vi "Tim Horizontal Bearing Control.vi"() -> ()   [LabVIEW 2020]
doc: "I. Description:\nThis example demonstrates how to output a single Voltage Update (Sample) to an Analog Output Channel.\n\nII. Instructions for Running:\n1. Select the Physical Channel to correspond to where your signal is output on the DAQ device.\n2. Enter the Minimum and Maximum Voltage Ranges\nNote: Use the Acq One Sample example to verify you are generating the correct output on the DAQ device\n\nIII. Block Diagram Steps:\n1. Create an Analog Output Voltage Channel\n2. Use the Write VI to Output 1 Sample to 1 Channel on the Data\nAcquisition Card. \n3. Call the Clear Task VI to clear the Task.\n4. Use the popup dialog box to display an error if any. \n\nIV. I/O Connections Overview:\nMake sure your signal output terminal matches the Physical Channel I/O Control. For further connection information, refer to your hardware reference manual."
uses:
  <vilib>/DAQmx/write.llb/DAQmx Write (Digital Bool 1Line 1Point).vi
  <vilib>/DAQmx/read.llb/DAQmx Read (Counter DBL 1Chan 1Samp).vi
  <extravilib>/ChannelInstances/Tag-bool/Write With Abort.vi
  <extravilib>/ChannelInstances/Tag-bool/Read With Abort.vi
  <extravilib>/ChannelInstances/Tag-dbl/Write With Abort.vi
  <extravilib>/ChannelInstances/Tag-dbl/Read With Abort.vi
  <vilib>/DAQmx/create/channels.llb/DAQmx Create Channel (CI-Frequency).vi
  <vilib>/DAQmx/configure/timing.llb/DAQmx Timing (Implicit).vi
  <vilib>/DAQmx/create/channels.llb/DAQmx Create Channel (DO-Digital Output).vi
  <extravilib>/ChannelInstances/Tag-bool/Instantiate.vi
  <extravilib>/ChannelInstances/Messenger-c(str,a[.](str),var)/Instantiate.vi
  <extravilib>/ChannelInstances/Tag-bool/Endpoint.vi
  <extravilib>/ChannelInstances/Tag-bool/EndpointRead.vi
  <extravilib>/ChannelInstances/Tag-dbl/Instantiate.vi
  <vilib>/DAQmx/miscellaneous.llb/DAQmx Fill In Error Info.vi
  <extravilib>/ChannelInstances/Tag-dbl/Endpoint.vi
  Labview_dependencies/channel_producer_dbl.vi
  <extravilib>/ChannelInstances/Tag-dbl/EndpointRead.vi
  <extravilib>/ChannelInstances/Tag-dbl.lvlib
  <extravilib>/ChannelInstances/Tag-bool.lvlib
  <resource>/objmgr/daqmx.rc
panel:
  in  "Relay":tag="cDAQ9189-horizontalMod7/port0/line5"
  in  "TCPIP Socket":refnum<visa-resource-name>="TCPIP0::10.0.0.52::5000::SOCKET"
  in  "CL Frequency Term":tag="/cDAQ9189-horizontalMod7/PFI0"
  in  "Counter":tag="cDAQ9189-horizontalMod7/ctr0"
  out "RPM":dbl
  in  "Toggle":bool
  in  "stop":bool
  in  "Save Folder":path
  in  "Save 2":bool
  out "Temp 1":dbl format="%.3f"
  out "Temp 2":dbl format="%.3f"
  out "Temp 3":dbl format="%.3f"
  out "Temp 4":dbl format="%.3f"
  out "Waveform Graph":dbl[][](graph)
  # "Physical Connections"
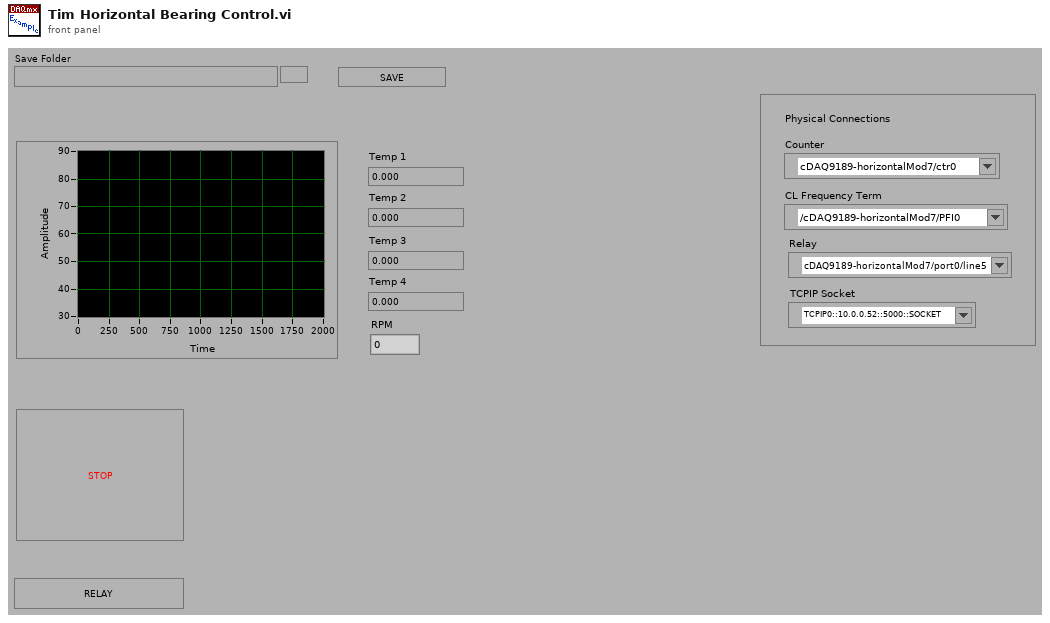
[diagram p1: front panel]
types:
  T1 = enum16{"open", "open or create", "create or replace", "create", "open (read-only)"}
  T2 = typedef "Tag-bool.lvlib/))Channel.ctl" = refnum<queue>
  T3 = typedef "Tag-dbl.lvlib/))Channel.ctl" = refnum<queue>
  T4 = typedef "Messenger-c(str,a[.](str),var).lvlib/))Channel.ctl" = refnum<queue>
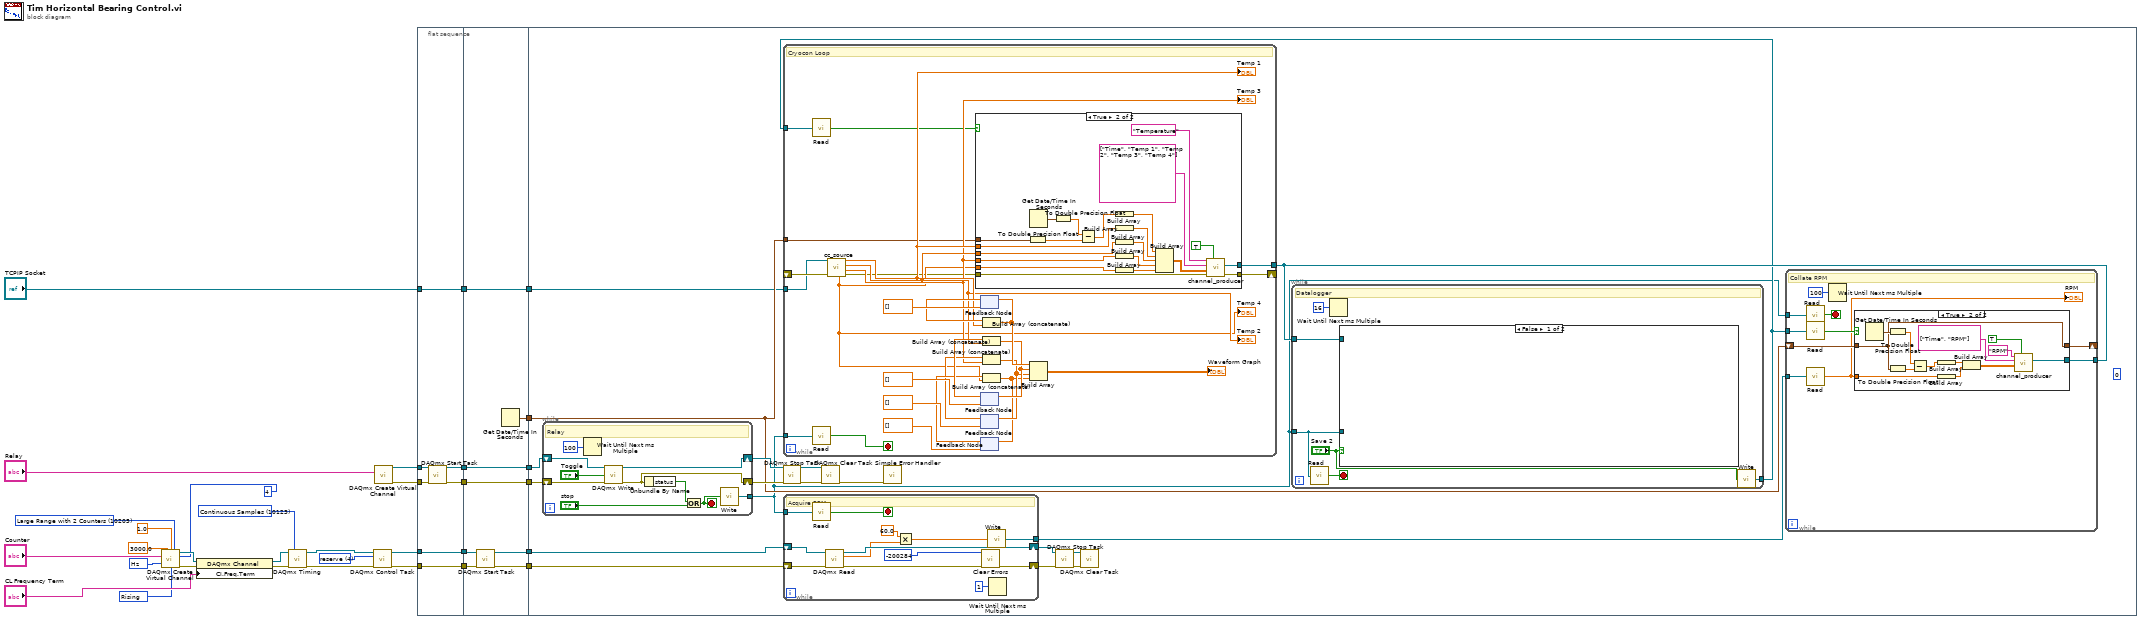
[diagram p0: block diagram]
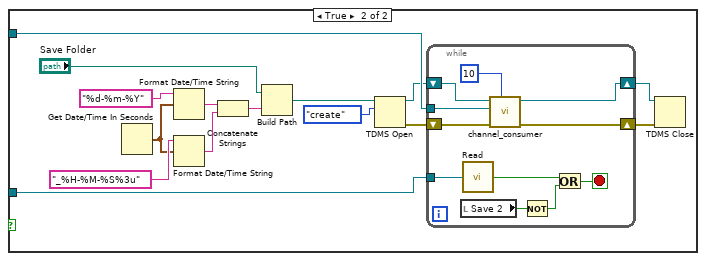
[diagram p3: hidden frame]
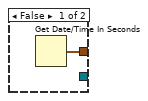
[diagram p4: hidden frame]
diagram:
  w3 = 10280 items=["Rising"=10280, "Falling"=10171] ("starting edge")
  w4 = 10373 items=["Hz"=10373, "Ticks"=10304, "From Custom Scale"=10065] ("units")
  w16 = 4 items=["verify"=2, "reserve"=4, "commit"=3, "unreserve"=5, "abort"=6] ("action")
  w14 = 10123 items=["Finite Samples"=10178, "Continuous Samples"=10123, "Hardware Timed Single Point"=12522] ("sample mode")
  w11 = 10205 items=["Low Frequency with 1 Counter"=10105, "High Frequency with 2 Counters"=10157, "Large Range with 2 Counters"=10205, "Dynamic Averaging"=16065] ("measurement method")
  n1 = call-poly <vilib>:"DAQmx Create Virtual Channel.vi"("maximum value"=3000.0, "minimum value"=1.0, "measurement method"=w11, "counter"="Counter", "divisor"=u32 4, "units"=w4, "starting edge"=w3) -> ("task out"=w17:refnum<k21>, "error out"=w18:errorcluster)  [unwired: 7 in]
  n2 = property class="DAQmx Channel"(reference=w17, error in=w18, "CI.Freq.Term"="CL Frequency Term") -> (reference out=w20:refnum<k21>, error out=w19:errorcluster)
  n3 = call-poly <vilib>:"DAQmx Timing.vi"("task/channels in"=w20, "sample mode"=w14, "error in"=w19) -> ("task out"=w21:refnum<k21>, "error out"=w22:errorcluster)  [unwired: 11 in]
  n4 = call <vilib>:"DAQmx Control Task.vi"("task/channels in"=w21, "action"=w16, "error in"=w22) -> ("task out"=w10:refnum<k21>, "error out"=w9:errorcluster)  [unwired: 11 in]
  n5 = call-poly <vilib>:"DAQmx Create Virtual Channel.vi"("lines"="Relay") -> ("task out"=w7:refnum<k21>, "error out"=w6:errorcluster)  [unwired: 13 in]
  n6 = flat-sequence {
    tunnel: [w40] -> w33
    tunnel: w10 -> [w40]
    tunnel: w9 -> [w39]
    tunnel: [w39] -> w32
    tunnel: [w38] -> w31
    tunnel: [w37] -> w30
    tunnel: w7 -> [w36]
    tunnel: w6 -> [w35]
    tunnel: "TCPIP Socket" -> [w34]
    tunnel: [w34] -> w29
    tunnel: [w48] -> w28
    tunnel: [w47] -> w27
    tunnel: [w46] -> w26
    tunnel: [w43] -> w25
    tunnel: [w42] -> w24
    tunnel: w33 -> [w45]
    tunnel: w32 -> [w44]
    tunnel: w31 -> [w43]
    tunnel: w30 -> [w42]
    tunnel: w29 -> [w41]
    tunnel: [w41] -> w23
    tunnel: w28 -> [w52]
    tunnel: w27 -> [w63]
    tunnel: w26 -> [w62]
    tunnel: w25 -> [w56]
    tunnel: w24 -> [w55]
    tunnel: w23 -> [w50]
    frame #0 {
      n7 = call <vilib>:"DAQmx Start Task.vi"("task/channels in"=w36, "error in"=w35) -> ("task out"=w38:refnum<k21>, "error out"=w37:errorcluster)  [unwired: 12 in]
    }
    frame #1 {
      n8 = call <vilib>:"DAQmx Start Task.vi"("task/channels in"=w45, "error in"=w44) -> ("task out"=w47:refnum<k21>, "error out"=w46:errorcluster)  [unwired: 12 in]
      n9 = Get Date/Time In Seconds() -> (seconds since 1Jan1904=w48:timestamp)
    }
    frame #2 {
      (unwired) 0
      n10 = while {
        shift-right: [w153] -> w57
        shift-left: w56 -> [w158]
        shift-right: [w152] -> w58
        shift-left: w55 -> [w157]
        tunnel: [w150] -> w49
        stop <- w149 stop-if-true
        # "Relay"
        n11 = Wait Until Next ms Multiple(millisecond multiple=u32 100) -> ()  [unwired: 1 out]
        n12 = call-poly <vilib>:"DAQmx Write.vi"("task/channels in"=w158, "data"="Toggle", "error in"=w157) -> ("task out"=w153:refnum<k21>, "error out"=w152:errorcluster)  [unwired: 10 in, 1 out]
        n13 = Unbundle By Name(w152) -> ("status"=w155:bool)
        n14 = Or(x=w155, y="stop") -> (x .or. y?=w149:bool)
        n15 = call <extravilib>:"Write.vi"("element"=w149) -> ("channel"=w150:T2)  [unwired: 1 out]
      }
      n16 = call <vilib>:"DAQmx Stop Task.vi"("task/channels in"=w57, "error in"=w58) -> ("task out"=w59:refnum<k21>, "error out"=w60:errorcluster)  [unwired: 12 in]
      n17 = while {
        shift-right: [w195] -> w64
        shift-left: w63 -> [w192]
        shift-right: [w186] -> w65
        shift-left: w62 -> [w191]
        tunnel: [w185] -> w61
        tunnel: w49 -> [w184]
        stop <- w183 stop-if-true
        # "Acquire RPM"
        n18 = call <extravilib>:"Read.vi"("channel"=w184) -> ("element"=w183:bool)  [unwired: 1 in, 1 out]
        n19 = call-poly <vilib>:"DAQmx Read.vi"("task/channels in"=w192, "error in"=w191) -> ("task out"=w195:refnum<k21>, "data"=w194:dbl, "error out"=w189:errorcluster)  [unwired: 11 in]
        n20 = Multiply(x=60.0, y=w194) -> (x*y=w187:dbl)
        n21 = call <vilib>:"Clear Errors.vi"("error in (no error)"=w189, "specific error code to clear (0: all)"=-200284) -> ("error out"=w186:errorcluster)  [unwired: 4 in, 1 out]
        n22 = call <extravilib>:"Write.vi"("element"=w187) -> ("channel"=w185:T3)  [unwired: 1 out]
        n23 = Wait Until Next ms Multiple(millisecond multiple=u32 1) -> ()  [unwired: 1 out]
      }
      n24 = call <vilib>:"DAQmx Clear Task.vi"("task in"=w59, "error in"=w60) -> ("error out"=w54:errorcluster)  [unwired: 13 in]
      n25 = call <vilib>:"Simple Error Handler.vi"("error in (no error)"=w54) -> ()  [unwired: 4 in, 5 out]
      n26 = call <vilib>:"DAQmx Stop Task.vi"("task/channels in"=w64, "error in"=w65) -> ("task out"=w67:refnum<k21>, "error out"=w66:errorcluster)  [unwired: 12 in]
      n27 = call <vilib>:"DAQmx Clear Task.vi"("task in"=w67, "error in"=w66) -> ()  [unwired: 13 in, 1 out]
      n28 = while {
        tunnel: w51 -> [w81]
        tunnel: w52 -> [w75]
        tunnel: [w74] -> w53
        tunnel: w49 -> [w73]
        shift-right: [w71] -> _
        shift-left: _ -> [w70]
        tunnel: w50 -> [w68]
        stop <- w69 stop-if-true
        # "Cryocon Loop"
        n29 = call <extravilib>:"Read.vi"("channel"=w81) -> ("element"=w76:bool)  [unwired: 1 in, 1 out]
        n30 = call <extravilib>:"Read.vi"("channel"=w73) -> ("element"=w69:bool)  [unwired: 1 in, 1 out]
        n31 = call "cc_source.vi"("error in (no error)"=w70, "VISA"=w68) -> ("Error Out"=w72:errorcluster, "Diode 3"=w78:dbl, "Diode 2"=w79:dbl, "Diode 1"=w80:dbl, "Diode 4"=w77:dbl)  [unwired: 5 in]
        "Temp 1" <- w80
        "Temp 2" <- w79
        "Temp 3" <- w78
        "Temp 4" <- w77
        n32 = case shown="True" w76 {
          tunnel: [_ w114] -> w74
          tunnel: w80 -> [_ w113]
          tunnel: w79 -> [_ w112]
          tunnel: w78 -> [_ w111]
          tunnel: w77 -> [_ w110]
          tunnel: w75 -> [_ w98]
          tunnel: w72 -> [w95 w97]
          tunnel: [w95 w96] -> w71
          frame False {
          }
          frame True {
            n33 = To Double Precision Float(number=w98) -> (double precision float=w104:dbl)
            n34 = Get Date/Time In Seconds() -> (seconds since 1Jan1904=w102:timestamp)
            n35 = To Double Precision Float(number=w102) -> (double precision float=w103:dbl)
            n36 = Subtract(x=w103, y=w104) -> (x-y=w101:dbl)
            n37 = Build Array(w101) -> (w99:dbl[])
            n38 = Build Array(w113) -> (w109:dbl[])
            n39 = Build Array(w112) -> (w108:dbl[])
            n40 = Build Array(w111) -> (w107:dbl[])
            n41 = Build Array(w110) -> (w106:dbl[])
            n42 = Build Array(w99, w109, w108, w107, w106) -> (w105:dbl[][])
            n43 = call-poly "channel_producer.vi"("Enable"=TRUE, "Error In"=w97, "Data"=w105, "Channels Names"=string[] ["Time", "Temp 1", "Temp 2", "Temp 3", "Temp 4"], "Group Name"="Temperature") -> ("Error Out"=w96:errorcluster, "TDMS Channel"=w114:T4)  [unwired: 2 in]
          }
        }
        n44 = feedback #1(dbl[] []) -> (w87:dbl[])
        n45 = feedback #2(dbl[] []) -> (w94:dbl[])
        n46 = feedback #3(dbl[] []) -> (w88:dbl[])
        n47 = feedback #4(dbl[] []) -> (w89:dbl[])
        n48 = Build Array (concatenate)(w87, w80) -> (w86:dbl[])
        n49 = feedback-in #1(w86) -> ()
        n50 = Build Array (concatenate)(w94, w79) -> (w85:dbl[])
        n51 = feedback-in #2(w85) -> ()
        n52 = Build Array (concatenate)(w88, w78) -> (w84:dbl[])
        n53 = feedback-in #3(w84) -> ()
        n54 = Build Array (concatenate)(w89, w77) -> (w83:dbl[])
        n55 = feedback-in #4(w83) -> ()
        n56 = Build Array(w86, w85, w84, w83) -> (→"Waveform Graph":dbl[][])
      }
      n57 = while {
        tunnel: w49 -> [w120]
        tunnel: w53 -> [w118]
        tunnel: [w117] -> w51
        stop <- w121 stop-if-true
        # "Datalogger"
        n58 = call <extravilib>:"Read.vi"("channel"=w120) -> ("element"=w121:bool)  [unwired: 1 in, 1 out]
        n59 = Wait Until Next ms Multiple(millisecond multiple=u32 16) -> ()  [unwired: 1 out]
        n60 = case shown="False" "Save 2" {
          tunnel: w120 -> [_ w129]
          tunnel: w118 -> [_ w127]
          frame False {
          }
          frame True {
            n61 = Get Date/Time In Seconds() -> (seconds since 1Jan1904=w134:timestamp)
            n62 = Format Date/Time String(time format string (%c)="%d-%m-%Y", seconds (now)=w134) -> (date/time string=w133:string)  [unwired: 1 in]
            n63 = Format Date/Time String(time format string (%c)="_%H-%M-%S%3u", seconds (now)=w134) -> (date/time string=w132:string)  [unwired: 1 in]
            n64 = Concatenate Strings(w133, w132) -> (w137:string)
            n65 = Build Path(base path="Save Folder", name or relative path=w137) -> (appended path=w130:path)
            n66 = TDMS Open(10:T1."create" ("operation (0:open)"), 11:w130) -> (0:w124:errorcluster, 3:w126:refnum<k34>)  [unwired: 5 in]
            n67 = while {
              tunnel: w129 -> [w148]
              tunnel: w127 -> [w142]
              shift-right: [w143] -> w125
              shift-left: w126 -> [w144]
              shift-right: [w140] -> w123
              shift-left: w124 -> [w141]
              stop <- w138 stop-if-true
              n68 = local read "Save 2"() -> (w146:bool)
              n69 = call <extravilib>:"Read.vi"("channel"=w148) -> ("element"=w147:bool)  [unwired: 1 in, 1 out]
              n70 = call "channel_consumer.vi"("timeout"=10, "error in"=w141, "TDMS channel"=w142, "TDMS in"=w144) -> ("error out"=w140:errorcluster, "TDMS out"=w143:refnum<k34>)  [unwired: 2 in, 1 out]
              n71 = Not(x=w146) -> (.not. x?=w145:bool)
              n72 = Or(x=w147, y=w145) -> (x .or. y?=w138:bool)
            }
            n73 = TDMS Close(8:w123, 11:w125) -> ()  [unwired: 2 out]
          }
        }
        n74 = call <extravilib>:"Write.vi"("element"="Save 2") -> ("channel"=w117:T2)  [unwired: 1 out]
      }
      n75 = while {
        tunnel: w61 -> [w168]
        tunnel: w53 -> [w163]
        tunnel: w51 -> [w162]
        tunnel: w49 -> [w160]
        shift-right: [w159] -> _
        shift-left: w52 -> [w166]
        stop <- w161 stop-if-true
        # "Collate RPM"
        n76 = call <extravilib>:"Read.vi"("channel"=w160) -> ("element"=w161:bool)  [unwired: 1 in, 1 out]
        n77 = call <extravilib>:"Read.vi"("channel"=w162) -> ("element"=w167:bool)  [unwired: 1 in, 1 out]
        n78 = call <extravilib>:"Read.vi"("channel"=w168) -> ("element"=w164:dbl)  [unwired: 1 in, 1 out]
        "RPM" <- w164
        n79 = Wait Until Next ms Multiple(millisecond multiple=u32 100) -> ()  [unwired: 1 out]
        n80 = case shown="True" w167 {
          tunnel: w166 -> [_ w170]
          tunnel: w164 -> [_ w172]
          tunnel: [_ w171] -> w163
          tunnel: [w169 w170] -> w159
          frame False {
            n81 = Get Date/Time In Seconds() -> (seconds since 1Jan1904=w169:timestamp)
          }
          frame True {
            n82 = Get Date/Time In Seconds() -> (seconds since 1Jan1904=w179:timestamp)
            n83 = To Double Precision Float(number=w179) -> (double precision float=w181:dbl)
            n84 = To Double Precision Float(number=w170) -> (double precision float=w180:dbl)
            n85 = Subtract(x=w181, y=w180) -> (x-y=w182:dbl)
            n86 = Build Array(w182) -> (w177:dbl[])
            n87 = Build Array(w172) -> (w176:dbl[])
            n88 = Build Array(w177, w176) -> (w175:dbl[][])
            n89 = call-poly "channel_producer.vi"("Enable"=TRUE, "Data"=w175, "Channels Names"=string[] ["Time", "RPM"], "Group Name"="RPM") -> ("TDMS Channel"=w171:T4)  [unwired: 3 in, 1 out]
          }
        }
      }
    }
  }
